vi "Navigation_florida_alex_rev0.vi"() -> ()   [LabVIEW 2015]
uses:
  <vilib>/myRIO/Instrument Drivers/Utilities/Utilities.lvlib
  <vilib>/rvi/interface/nirviReadWriteControl/nirviReadWriteControl.xnode
  NiFpgaLv.dll
  <vilib>/Utility/error.llb/Error Cluster From Error Code.vi
  <vilib>/rvi/interface/Simulation/niFpgaSimulationCallBeginRW.vi
  <vilib>/rvi/errors/niLvFpgaAdjustHostInterfaceError.vi
  <vilib>/rvi/interface/nirviOpenFPGA/nirviOpenFPGA.xnode
  FPGA Bitfiles/NavigationProjec_FPGATarget2_FPGAMainNavigati_PWPHW8gwDxI.lvbitx
  <vilib>/FPGAPlugInAG/myRIO-1900/niLvFpga_Open_myRIO-1900.vi
  <vilib>/rvi/interface/common/dynamic/niFpgaDynamicAddResources.vi
  <vilib>/myRIO/Instrument Drivers/Onboard IO/PWM/typedefs/PWM Configuration.ctl
  <vilib>/myRIO/Instrument Drivers/Onboard IO/PWM/PWM.lvlib
  <vilib>/myRIO/Common/Instrument Driver Framework/myRIO v1.0/PWM/typedefs/PWM Channels Enum.ctl
  <vilib>/myRIO/Common/Instrument Driver Framework/Utilities/typedefs/Generic FPGA Reference.ctl
  <vilib>/myRIO/Common/Instrument Driver Framework/Utilities/typedefs/myRIO v1.0 Reference.ctl
  <vilib>/myRIO/Common/Instrument Driver Framework/Utilities/typedefs/Hardware Version Enum.ctl
  <vilib>/myRIO/Common/Instrument Driver Framework/Utilities/typedefs/myRIO Generic Hardware Reference.ctl
  <vilib>/myRIO/Instrument Drivers/Onboard IO/PWM/typedefs/PWM Reference.ctl
  <vilib>/myRIO/Instrument Drivers/Onboard IO/PWM/vis/myRIO PWM Open.xnode
  <vilib>/myRIO/Common/Instrument Driver Framework/myRIO v1.0/PWM/vis/myRIO v1.1 Open PWM.vi
  <vilib>/userdefined/High Color/nirio_resource_hc.ctl
  <vilib>/addons/control/pid/NI_PID_pid.lvlib
  <vilib>/addons/control/pid/pid.llb/PID (DBL).vi
panel:
  in  "PID Gains Right":T1={"proportional gain (Kc)"=1.0, "integral time (Ti, min)"=0.01, "derivative time (Td, min)"=0.0} {"derivative time (Td, min)" format="%.3f"; "integral time (Ti, min)" format="%.3f"; "proportional gain (Kc)" format="%.3f"}
  in  "Output Range Right":cluster{"output high":dbl, "output low":dbl}={"output high"=100.0, "output low"=-100.0} {"output low" format="%.2f"; "output high" format="%.2f"}
  in  "Output Range Left":cluster{"output high":dbl, "output low":dbl}={"output high"=100.0, "output low"=-100.0} {"output low" format="%.2f"; "output high" format="%.2f"}
  in  "PID Gains Left":T1={"proportional gain (Kc)"=1.0, "integral time (Ti, min)"=0.01, "derivative time (Td, min)"=0.0} {"derivative time (Td, min)" format="%.3f"; "integral time (Ti, min)" format="%.3f"; "proportional gain (Kc)" format="%.3f"}
  out "Right Setpoint":dbl
  out "Left Setpoint":dbl
  out "Scale":dbl
  out "Distance to Goal":dbl
  out "Current Angle":dbl
  out "Current Y":dbl
  out "Current X":dbl
  out "State":i32
  out "Dump Angle":dbl
  out "Dump Y":dbl
  out "Dump X":dbl
  out "Start Case":i32
  out "Goal Y":dbl
  out "Goal X":dbl
  out "Start Angle":dbl
  out "Start Y":dbl
  out "Start X":dbl
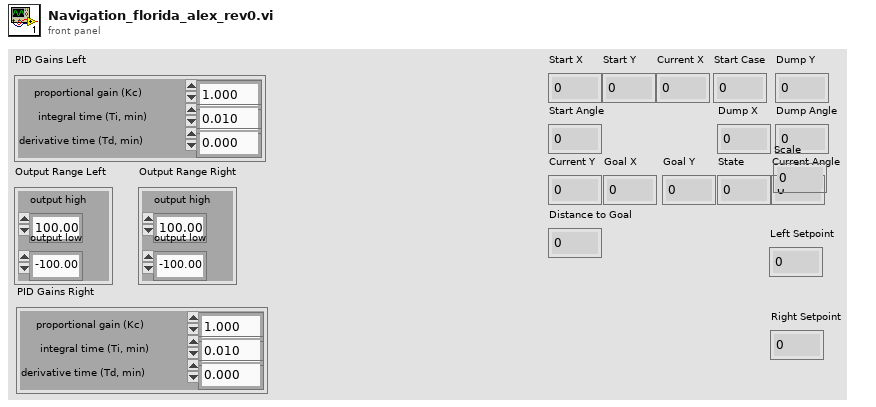
[diagram p1: front panel]
types:
  T1 = cluster{"proportional gain (Kc)":dbl, "integral time (Ti, min)":dbl, "derivative time (Td, min)":dbl}
  T2 = typedef "nirio_resource_hc.ctl" = tag
  T3 = typedef "Hardware Version Enum.ctl" = enum16{"Unknown", "myRIO-1900", "myRIO-1950", "roboRIO"}
  T4 = typedef "PWM.lvlib/PWM Reference.ctl" = cluster{"myRIO Reference":T5, "PWM Channels Enum":T8, "PWM Configuration":T9}
  T5 = typedef "myRIO Generic Hardware Reference.ctl" = cluster{"myRIO Model":T3, "myRIO Hardware Reference":T6}
  T6 = typedef "myRIO v1.0 Reference.ctl" = cluster{"Generic FPGA Reference":T7, "Allow multiple opens":bool}
  T7 = typedef "Generic FPGA Reference.ctl" = refnum<k20>
  T8 = typedef "PWM Channels Enum.ctl" = enum16{"Not Connected", "C/PWM0", "C/PWM1", "A/PWM0", "A/PWM1", "A/PWM2", "B/PWM0", "B/PWM1", "B/PWM2", "PWM/PWM0", "PWM/PWM1", "PWM/PWM2", "PWM/PWM3", "PWM/PWM4", "PWM/PWM5", "PWM/PWM6", "PWM/PWM7", "PWM/PWM8", "PWM/PWM9"}
  T9 = typedef "PWM.lvlib/PWM Configuration.ctl" = cluster{"Frequency":dbl, "Duty Cycle":dbl}
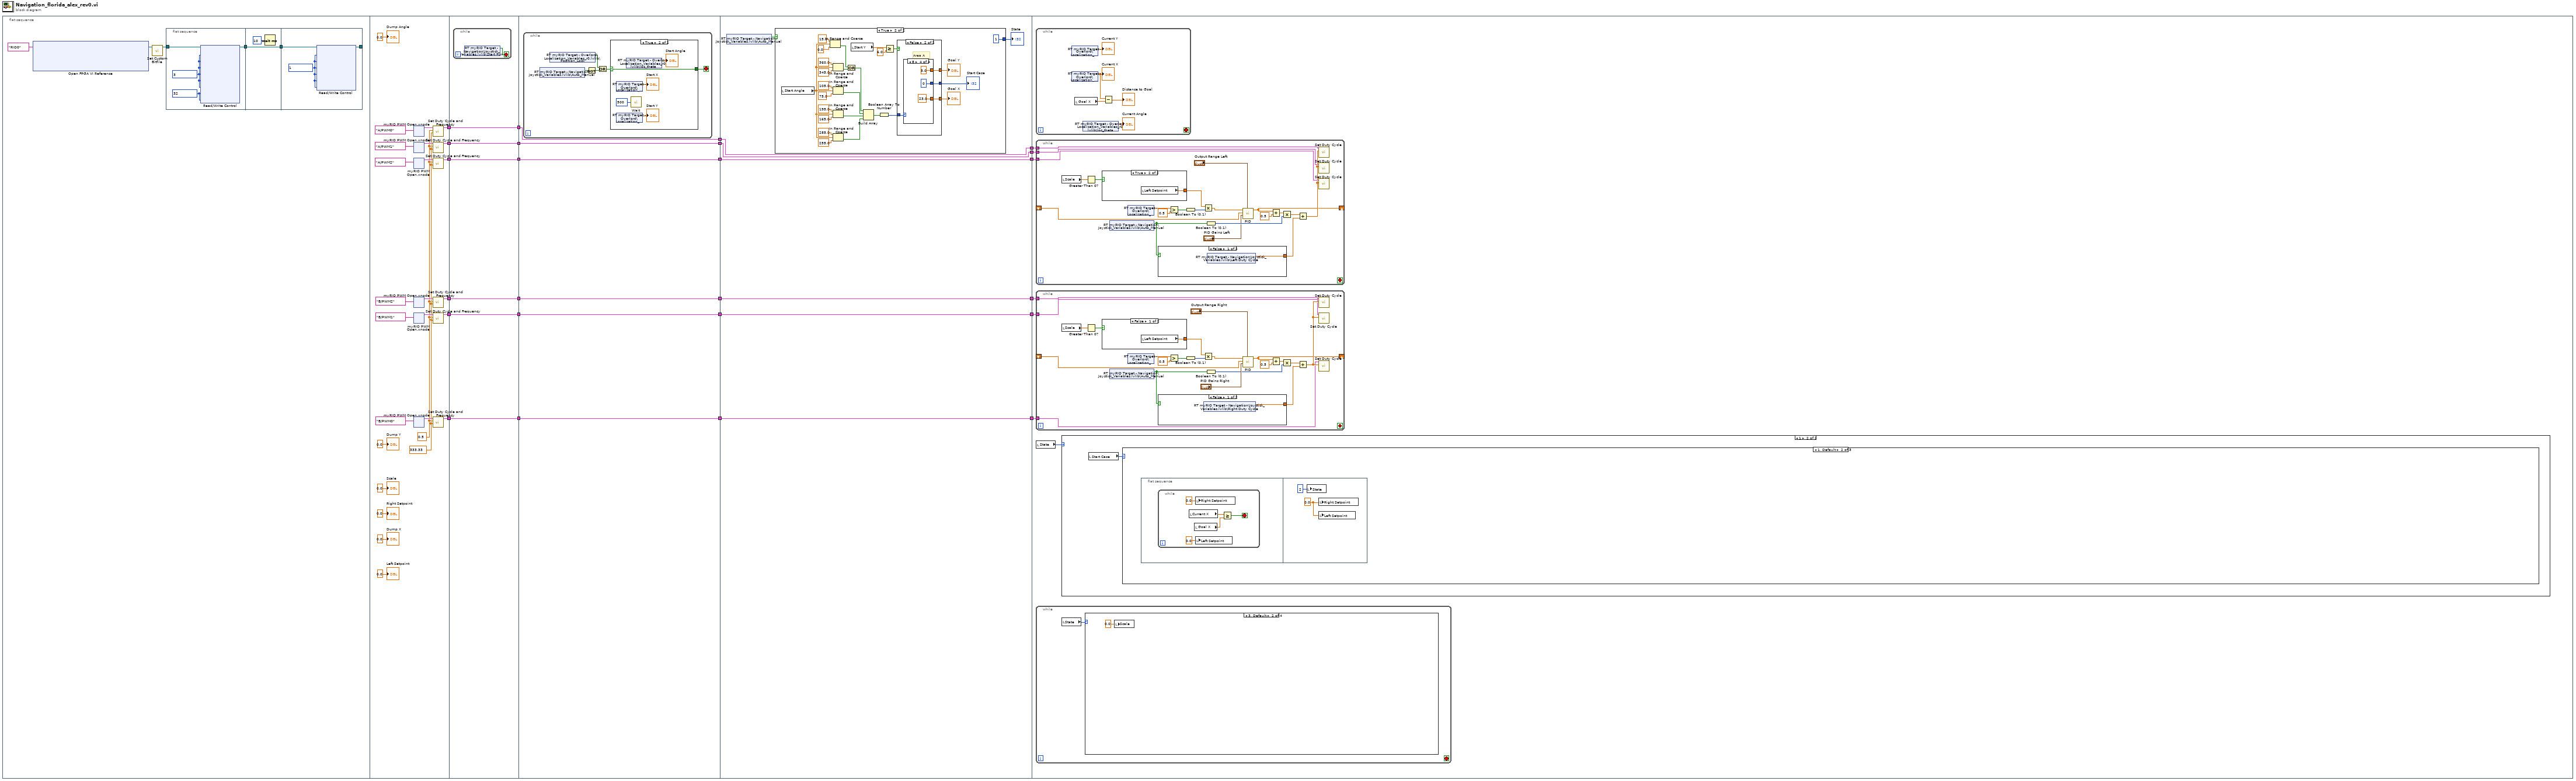
[diagram p0: block diagram]
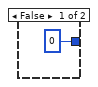
[diagram p3: hidden frame]
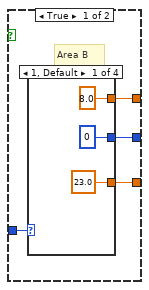
[diagram p4: hidden frame]
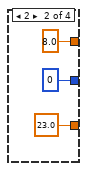
[diagram p5: hidden frame]
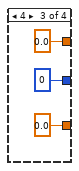
[diagram p6: hidden frame]
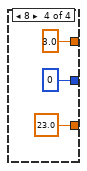
[diagram p7: hidden frame]
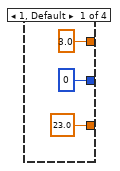
[diagram p8: hidden frame]
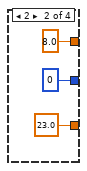
[diagram p9: hidden frame]
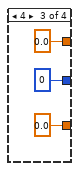
[diagram p10: hidden frame]
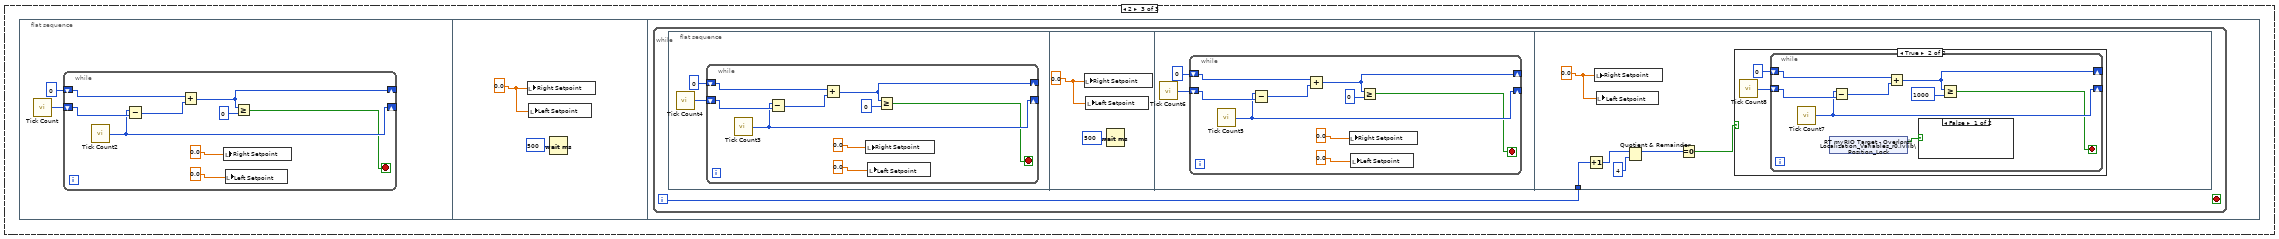
[diagram p13: hidden frame]
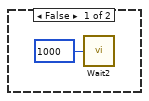
[diagram p14: hidden frame]
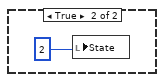
[diagram p15: hidden frame]
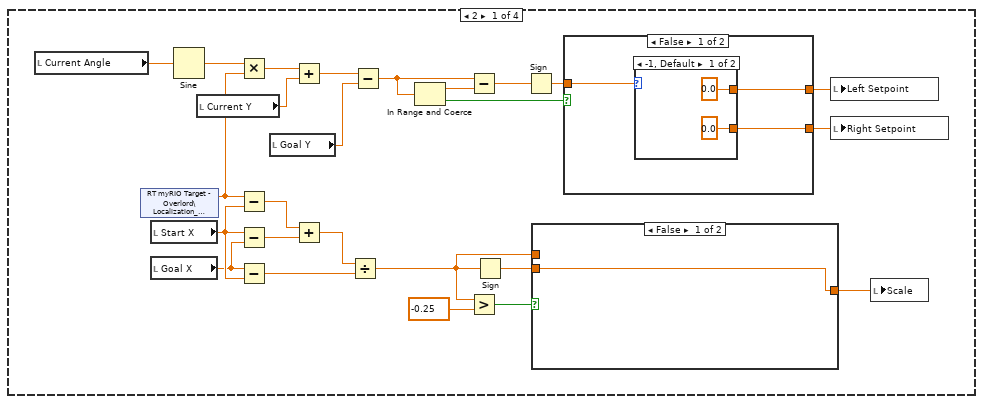
[diagram p16: hidden frame]
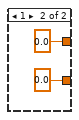
[diagram p17: hidden frame]
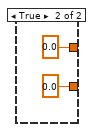
[diagram p18: hidden frame]
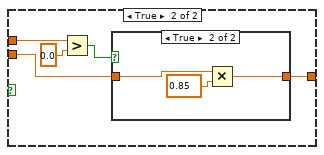
[diagram p19: hidden frame]
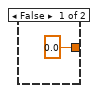
[diagram p20: hidden frame]
diagram:
  n1 = flat-sequence {
    tunnel: [w50] -> w24
    tunnel: [w49] -> w23
    tunnel: [w48] -> w22
    tunnel: [w47] -> w21
    tunnel: [w46] -> w20
    tunnel: [w45] -> w19
    tunnel: w24 -> [w166]
    tunnel: w23 -> [w165]
    tunnel: w22 -> [w164]
    tunnel: w21 -> [w163]
    tunnel: w20 -> [w162]
    tunnel: w19 -> [w161]
    tunnel: [w166] -> w18
    tunnel: [w165] -> w17
    tunnel: [w164] -> w16
    tunnel: [w163] -> w15
    tunnel: [w162] -> w14
    tunnel: [w161] -> w13
    tunnel: w18 -> [w173]
    tunnel: w17 -> [w172]
    tunnel: w16 -> [w171]
    tunnel: w15 -> [w170]
    tunnel: w14 -> [w169]
    tunnel: w13 -> [w168]
    tunnel: [w173] -> w12
    tunnel: [w172] -> w11
    tunnel: [w171] -> w10
    tunnel: [w170] -> w9
    tunnel: [w169] -> w8
    tunnel: [w168] -> w7
    tunnel: w12 -> [w192]
    tunnel: w11 -> [w191]
    tunnel: w10 -> [w190]
    tunnel: w9 -> [w189]
    tunnel: w8 -> [w188]
    tunnel: w7 -> [w187]
    tunnel: [w192] -> w6
    tunnel: [w191] -> w5
    tunnel: [w190] -> w4
    tunnel: [w189] -> w3
    tunnel: [w188] -> w2
    tunnel: [w187] -> w1
    tunnel: w6 -> [w258]
    tunnel: w5 -> [w257]
    tunnel: w4 -> [w256]
    tunnel: w3 -> [w255]
    tunnel: w2 -> [w254]
    tunnel: w1 -> [w253]
    frame #0 {
      n2 = xnode "Open FPGA VI Reference"("resource name"=tag "RIO0") -> ("FPGA VI Reference Out"=w26:refnum<k20>)  [unwired: 1 in, 1 out]
      n3 = call <vilib>:"Set Custom Bitfile.vi"("Custom FPGA Reference In"=w26) -> ("Custom FPGA Reference Out"=w27:refnum<k20>)  [unwired: 9 in, 1 out]
      n4 = flat-sequence {
        tunnel: w27 -> [w32]
        tunnel: [w30] -> w29
        tunnel: w29 -> [w34]
        tunnel: [w34] -> w28
        tunnel: w28 -> [w37]
        tunnel: [w36] -> _
        frame #0 {
          w31 = u8 32 ("SYS.SELECTA")
          w33 = u8 3 ("ENC.B_c.CNFG")
          n5 = xnode "Read/Write Control"("FPGA VI Reference In"=w32, "ENC.A_a.CNFG"=w33, "ENC.A_b.CNFG"=w33, "ENC.A_c.CNFG"=w33, "ENC.B_a.CNFG"=w33, "ENC.B_b.CNFG"=w33, "ENC.B_c.CNFG"=w33, "SYS.SELECTA"=w31, "SYS.SELECTB"=w31) -> ("FPGA VI Reference Out"=w30:refnum<k20>)  [unwired: 1 in, 1 out]
        }
        frame #1 {
          n6 = Wait (ms)(milliseconds to wait=u32 10) -> ()  [unwired: 1 out]
        }
        frame #2 {
          w38 = u8 1 ("ENC.B_c.CNFG")
          n7 = xnode "Read/Write Control"("FPGA VI Reference In"=w37, "ENC.A_a.CNFG"=w38, "ENC.A_b.CNFG"=w38, "ENC.A_c.CNFG"=w38, "ENC.B_a.CNFG"=w38, "ENC.B_b.CNFG"=w38, "ENC.B_c.CNFG"=w38) -> ("FPGA VI Reference Out"=w36:refnum<k20>)  [unwired: 1 in, 1 out]
        }
      }
    }
    frame #1 {
      w51 = 0.5
      w52 = 333.33
      n8 = xnode "myRIO PWM Open.xnode"("Channel Name"=tag "A/PWM0") -> ("PWM Ref Out"=w58:T4)  [unwired: 2 in, 1 out]
      n9 = xnode "myRIO PWM Open.xnode"("Channel Name"=tag "A/PWM1") -> ("PWM Ref Out"=w57:T4)  [unwired: 2 in, 1 out]
      n10 = xnode "myRIO PWM Open.xnode"("Channel Name"=tag "A/PWM2") -> ("PWM Ref Out"=w56:T4)  [unwired: 2 in, 1 out]
      n11 = xnode "myRIO PWM Open.xnode"("Channel Name"=tag "B/PWM2") -> ("PWM Ref Out"=w53:T4)  [unwired: 2 in, 1 out]
      n12 = xnode "myRIO PWM Open.xnode"("Channel Name"=tag "B/PWM1") -> ("PWM Ref Out"=w54:T4)  [unwired: 2 in, 1 out]
      n13 = xnode "myRIO PWM Open.xnode"("Channel Name"=tag "B/PWM0") -> ("PWM Ref Out"=w55:T4)  [unwired: 2 in, 1 out]
      n14 = call <vilib>:"Set Duty Cycle and Frequency.vi"("Frequency [Hz]"=w52, "Duty Cycle"=w51, "PWM Ref In"=w58) -> ("PWM Ref Out"=w50:T4)  [unwired: 6 in, 1 out]
      n15 = call <vilib>:"Set Duty Cycle and Frequency.vi"("Frequency [Hz]"=w52, "Duty Cycle"=w51, "PWM Ref In"=w57) -> ("PWM Ref Out"=w49:T4)  [unwired: 6 in, 1 out]
      n16 = call <vilib>:"Set Duty Cycle and Frequency.vi"("Frequency [Hz]"=w52, "Duty Cycle"=w51, "PWM Ref In"=w56) -> ("PWM Ref Out"=w48:T4)  [unwired: 6 in, 1 out]
      n17 = call <vilib>:"Set Duty Cycle and Frequency.vi"("Frequency [Hz]"=w52, "Duty Cycle"=w51, "PWM Ref In"=w53) -> ("PWM Ref Out"=w45:T4)  [unwired: 6 in, 1 out]
      n18 = call <vilib>:"Set Duty Cycle and Frequency.vi"("Frequency [Hz]"=w52, "Duty Cycle"=w51, "PWM Ref In"=w54) -> ("PWM Ref Out"=w46:T4)  [unwired: 6 in, 1 out]
      n19 = call <vilib>:"Set Duty Cycle and Frequency.vi"("Frequency [Hz]"=w52, "Duty Cycle"=w51, "PWM Ref In"=w55) -> ("PWM Ref Out"=w47:T4)  [unwired: 6 in, 1 out]
      "Dump X" <- 0.0
      "Dump Y" <- 0.0
      "Dump Angle" <- 0.0
      "Scale" <- 0.0
      "Left Setpoint" <- 0.0
      "Right Setpoint" <- 0.0
    }
    frame #2 {
      n20 = while {
        stop <- w167 stop-if-true
        n21 = shared-variable "RT myRIO Target - Navigation\\Joystick_Variables.lvlib\\Start Run"() -> (w167:bool)  [unwired: 1 in, 1 out]
      }
    }
    frame #3 {
      n22 = while {
        stop <- w174 stop-if-true
        n23 = shared-variable "RT myRIO Target - Navigation\\Joystick_Variables.lvlib\\Auto_Manual"() -> (w177:bool)  [unwired: 1 in, 1 out]
        n24 = shared-variable "RT myRIO Target - Overlord\\Localization_Variables_r0.lvlib\\Position_Lock"() -> (w178:bool)  [unwired: 1 in, 1 out]
        n25 = Not(x=w177) -> (.not. x?=w176:bool)
        n26 = Or(x=w178, y=w176) -> (x .or. y?=w175:bool)
        n27 = case shown="True" w175 {
          selector: w175 -> [w179 w181]
          tunnel: [w179 w181] -> w174
          frame False {
          }
          frame True {
            n28 = shared-variable "RT myRIO Target - Overlord\\Localization_Variables_r0.lvlib\\loc_x"() -> (→"Start X":dbl)  [unwired: 1 in, 1 out]
            n29 = shared-variable "RT myRIO Target - Overlord\\Localization_Variables_r0.lvlib\\loc_y"() -> (→"Start Y":dbl)  [unwired: 1 in, 1 out]
            n30 = shared-variable "RT myRIO Target - Overlord\\Localization_Variables_r0.lvlib\\loc_theta"() -> (→"Start Angle":dbl)  [unwired: 1 in, 1 out]
            n31 = call "Wait"("Count(mSec)"=u32 500) -> ()  [unwired: 1 out]
          }
        }
      }
    }
    frame #4 {
      n32 = shared-variable "RT myRIO Target - Navigation\\Joystick_Variables.lvlib\\Auto_Manual"() -> (w186:bool)  [unwired: 1 in, 1 out]
      n33 = case shown="True" w186 {
        tunnel: [0 1] -> w185
        frame False {
        }
        frame True {
          n34 = local read "Start Angle"() -> (w206:dbl)
          n35 = In Range and Coerce(upper limit=15.0, x=w206, lower limit=0.0) -> (In Range?=w205:bool)  [unwired: 1 out]
          n36 = In Range and Coerce(upper limit=360.0, x=w206, lower limit=345.0) -> (In Range?=w204:bool)  [unwired: 1 out]
          n37 = In Range and Coerce(upper limit=105.0, x=w206, lower limit=75.0) -> (In Range?=w202:bool)  [unwired: 1 out]
          n38 = In Range and Coerce(upper limit=195.0, x=w206, lower limit=165.0) -> (In Range?=w201:bool)  [unwired: 1 out]
          n39 = In Range and Coerce(upper limit=285.0, x=w206, lower limit=255.0) -> (In Range?=w200:bool)  [unwired: 1 out]
          n40 = Or(x=w205, y=w204) -> (x .or. y?=w203:bool)
          n41 = local read "Start Y"() -> (w219:dbl)
          n42 = Build Array(w203, w202, w201, w200) -> (w199:bool[])
          n43 = Boolean Array To Number(Boolean array=w199) -> (number=w198:u32)
          n44 = Greater Or Equal?(x=w219, y=6.0) -> (x >= y?=w217:bool)
          n45 = case shown="False" w217 {
            tunnel: w198 -> [w223 w239]
            tunnel: [w222 w238] -> w197
            tunnel: [w221 w237] -> w196
            tunnel: [w220 w236] -> w195
            frame True {
              # "Area B"
              n46 = case shown="1, Default" w223 {
                tunnel: [0 0 0 0] -> w220
                tunnel: [8.0 8.0 0.0 3.0] -> w221
                tunnel: [23.0 23.0 0.0 23.0] -> w222
                frame 1, Default {
                }
                frame 2 {
                }
                frame 4 {
                }
                frame 8 {
                }
              }
            }
            frame False {
              # "Area A"
              n47 = case shown="8" w239 {
                tunnel: [0 0 0 0] -> w236
                tunnel: [3.0 8.0 0.0 3.0] -> w237
                tunnel: [23.0 23.0 0.0 23.0] -> w238
                frame 1, Default {
                }
                frame 2 {
                }
                frame 4 {
                }
                frame 8 {
                }
              }
            }
          }
          "Goal X" <- w197
          "Goal Y" <- w196
          "Start Case" <- w195
        }
      }
      "State" <- w185
    }
    frame #5 {
      n48 = while {
        stop <- _ stop-if-true
        n49 = shared-variable "RT myRIO Target - Overlord\\Localization_Variables_r0.lvlib\\loc_y"() -> (→"Current Y":dbl)  [unwired: 1 in, 1 out]
        n50 = shared-variable "RT myRIO Target - Overlord\\Localization_Variables_r0.lvlib\\loc_x"() -> (w468:dbl)  [unwired: 1 in, 1 out]
        "Current X" <- w468
        n51 = local read "Goal X"() -> (w467:dbl)
        n52 = shared-variable "RT myRIO Target - Overlord\\Localization_Variables_r0.lvlib\\loc_theta"() -> (→"Current Angle":dbl)  [unwired: 1 in, 1 out]
        n53 = Subtract(x=w468, y=w467) -> (x-y=→"Distance to Goal":dbl)
      }
      n54 = while {
        tunnel: w258 -> [w447]
        tunnel: w257 -> [w446]
        tunnel: w256 -> [w445]
        shift-right: [w443] -> _
        shift-left: _ -> [w442]
        stop <- _ stop-if-true
        n55 = local read "Scale"() -> (w461:dbl)
        n56 = Greater Than 0?(x=w461) -> (x > 0?=w460:bool)
        n57 = case shown="True" w460 {
          tunnel: [w464 w465] -> w455
          frame False {
            n58 = local read "Right Setpoint"() -> (w464:dbl)
          }
          frame True {
            n59 = local read "Left Setpoint"() -> (w465:dbl)
          }
        }
        n60 = shared-variable "RT myRIO Target - Navigation\\Joystick_Variables.lvlib\\Auto_Manual"() -> (w459:bool)  [unwired: 1 in, 1 out]
        n61 = shared-variable "RT myRIO Target - Overlord\\Localization_Variables_r0.lvlib\\loc_x"() -> (w458:dbl)  [unwired: 1 in, 1 out]
        n62 = case shown="False" w459 {
          tunnel: [w462 0.0] -> w449
          frame False {
            n63 = shared-variable "RT myRIO Target - Navigation\\Joystick_Variables.lvlib\\Left Duty Cycle"() -> (w462:dbl)  [unwired: 1 in, 1 out]
          }
          frame True {
          }
        }
        n64 = Greater?(x=w458, y=0.5) -> (0:w456:bool)
        n65 = Boolean To (0,1)(Boolean=w456) -> (0, 1=w454:i16)
        n66 = Multiply(x=w455, y=w454) -> (x*y=w453:dbl)
        n67 = Boolean To (0,1)(Boolean=w459) -> (0, 1=w452:i16)
        n68 = call-poly <vilib>:"PID.vi"("output range"="Output Range Left", "PID gains"="PID Gains Left", "process variable"=w442, "setpoint"=w453) -> ("output"=w443:dbl)  [unwired: 6 in, 1 out]
        n69 = Add(x=w443, y=0.5) -> (x+y=w450:dbl)
        n70 = Multiply(x=w450, y=w452) -> (x*y=w448:dbl)
        n71 = Add(x=w448, y=w449) -> (x+y=w444:dbl)
        n72 = call <vilib>:"Set Duty Cycle.vi"("Duty Cycle"=w444, "PWM Ref In"=w447) -> ()  [unwired: 7 in, 2 out]
        n73 = call <vilib>:"Set Duty Cycle.vi"("Duty Cycle"=w444, "PWM Ref In"=w446) -> ()  [unwired: 7 in, 2 out]
        n74 = call <vilib>:"Set Duty Cycle.vi"("Duty Cycle"=w444, "PWM Ref In"=w445) -> ()  [unwired: 7 in, 2 out]
      }
      n75 = while {
        tunnel: w255 -> [w418]
        tunnel: w254 -> [w417]
        tunnel: w253 -> [w416]
        shift-right: [w415] -> _
        shift-left: _ -> [w414]
        stop <- _ stop-if-true
        n76 = local read "Scale"() -> (w435:dbl)
        n77 = Greater Than 0?(x=w435) -> (x > 0?=w434:bool)
        n78 = case shown="False" w434 {
          tunnel: [w438 w439] -> w430
          frame False {
            n79 = local read "Left Setpoint"() -> (w438:dbl)
          }
          frame True {
            n80 = local read "Right Setpoint"() -> (w439:dbl)
          }
        }
        n81 = shared-variable "RT myRIO Target - Navigation\\Joystick_Variables.lvlib\\Auto_Manual"() -> (w428:bool)  [unwired: 1 in, 1 out]
        n82 = shared-variable "RT myRIO Target - Overlord\\Localization_Variables_r0.lvlib\\loc_x"() -> (w431:dbl)  [unwired: 1 in, 1 out]
        n83 = case shown="False" w428 {
          tunnel: [w436 0.0] -> w420
          frame False {
            n84 = shared-variable "RT myRIO Target - Navigation\\Joystick_Variables.lvlib\\Right Duty Cycle"() -> (w436:dbl)  [unwired: 1 in, 1 out]
          }
          frame True {
          }
        }
        n85 = Greater?(x=w431, y=0.5) -> (0:w433:bool)
        n86 = Boolean To (0,1)(Boolean=w433) -> (0, 1=w429:i16)
        n87 = Multiply(x=w430, y=w429) -> (x*y=w427:dbl)
        n88 = Boolean To (0,1)(Boolean=w428) -> (0, 1=w422:i16)
        n89 = call-poly <vilib>:"PID.vi"("output range"="Output Range Right", "PID gains"="PID Gains Right", "process variable"=w414, "setpoint"=w427) -> ("output"=w415:dbl)  [unwired: 6 in, 1 out]
        n90 = Add(x=w415, y=0.5) -> (x+y=w423:dbl)
        n91 = Multiply(x=w423, y=w422) -> (x*y=w421:dbl)
        n92 = Add(x=w421, y=w420) -> (x+y=w419:dbl)
        n93 = call <vilib>:"Set Duty Cycle.vi"("Duty Cycle"=w419, "PWM Ref In"=w416) -> ()  [unwired: 7 in, 2 out]
        n94 = call <vilib>:"Set Duty Cycle.vi"("Duty Cycle"=w419, "PWM Ref In"=w417) -> ()  [unwired: 7 in, 2 out]
        n95 = call <vilib>:"Set Duty Cycle.vi"("Duty Cycle"=w419, "PWM Ref In"=w418) -> ()  [unwired: 7 in, 2 out]
      }
      n96 = local read "State"() -> (w252:i32)
      n97 = while {
        stop <- _ stop-if-true
        n98 = local read "State"() -> (w323:i32)
        n99 = case shown="3, Default" w323 {
          frame 2 {
            n100 = local read "Current Angle"() -> (w337:dbl)
            n101 = shared-variable "RT myRIO Target - Overlord\\Localization_Variables_r0.lvlib\\loc_x"() -> (w335:dbl)  [unwired: 1 in, 1 out]
            n102 = local read "Start X"() -> (w348:dbl)
            n103 = local read "Goal X"() -> (w347:dbl)
            n104 = Sine(x=w337) -> (sin(x)=w336:dbl)
            n105 = local read "Current Y"() -> (w333:dbl)
            n106 = Multiply(x=w336, y=w335) -> (x*y=w334:dbl)
            n107 = Subtract(x=w335, y=w348) -> (x-y=w346:dbl)
            n108 = Subtract(x=w348, y=w347) -> (x-y=w345:dbl)
            n109 = Subtract(x=w347, y=w348) -> (x-y=w344:dbl)
            n110 = local read "Goal Y"() -> (w332:dbl)
            n111 = Add(x=w334, y=w333) -> (x+y=w331:dbl)
            n112 = Add(x=w346, y=w345) -> (x+y=w343:dbl)
            n113 = Divide(x=w343, y=w344) -> (x/y=w340:dbl)
            n114 = Subtract(x=w331, y=w332) -> (x-y=w328:dbl)
            n115 = In Range and Coerce(x=w328) -> (coerced(x)=w329:dbl, In Range?=w330:bool)  [unwired: 2 in]
            n116 = Subtract(x=w328, y=w329) -> (x-y=w327:dbl)
            n117 = Greater?(x=w340, y=-0.25) -> (0:w341:bool)
            n118 = Sign(1:w340) -> (0:w339:dbl)
            n119 = Sign(1:w327) -> (0:w326:dbl)
            n120 = case shown="False" w341 {
              tunnel: w340 -> [_ w362]
              tunnel: w339 -> [w358 w360]
              tunnel: [w358 w359] -> w338
              frame False {
              }
              frame True {
                n121 = Greater?(x=w362, y=0.0) -> (0:w361:bool)
                n122 = case shown="True" w361 {
                  tunnel: w360 -> [_ w367]
                  tunnel: [0.0 w365] -> w359
                  frame False {
                  }
                  frame True {
                    n123 = Multiply(x=w367, y=0.85) -> (x*y=w365:dbl)
                  }
                }
              }
            }
            n124 = case shown="False" w330 {
              tunnel: w326 -> [w351 _]
              tunnel: [w350 0.0] -> w324
              tunnel: [w349 0.0] -> w325
              frame False {
                n125 = case shown="-1, Default" w351 {
                  tunnel: [0.0 0.0] -> w350
                  tunnel: [0.0 0.0] -> w349
                  frame -1, Default {
                  }
                  frame 1 {
                  }
                }
              }
              frame True {
              }
            }
            n126 = local write "Left Setpoint"(w325) -> ()
            n127 = local write "Right Setpoint"(w324) -> ()
            n128 = local write "Scale"(w338) -> ()
          }
          frame 3, Default {
            n129 = local write "Scale"(0.0) -> ()
          }
          frame 4 {
            n130 = local read "Current Angle"() -> (w382:dbl)
            n131 = shared-variable "RT myRIO Target - Overlord\\Localization_Variables_r0.lvlib\\loc_x"() -> (w380:dbl)  [unwired: 1 in, 1 out]
            n132 = local read "Start X"() -> (w393:dbl)
            n133 = local read "Goal X"() -> (w392:dbl)
            n134 = Sine(x=w382) -> (sin(x)=w381:dbl)
            n135 = local read "Current Y"() -> (w378:dbl)
            n136 = Multiply(x=w381, y=w380) -> (x*y=w379:dbl)
            n137 = Subtract(x=w380, y=w393) -> (x-y=w391:dbl)
            n138 = Subtract(x=w393, y=w392) -> (x-y=w390:dbl)
            n139 = Subtract(x=w392, y=w393) -> (x-y=w389:dbl)
            n140 = local read "Goal Y"() -> (w377:dbl)
            n141 = Add(x=w379, y=w378) -> (x+y=w376:dbl)
            n142 = Add(x=w391, y=w390) -> (x+y=w388:dbl)
            n143 = Divide(x=w388, y=w389) -> (x/y=w385:dbl)
            n144 = Subtract(x=w376, y=w377) -> (x-y=w373:dbl)
            n145 = In Range and Coerce(x=w373) -> (coerced(x)=w374:dbl, In Range?=w375:bool)  [unwired: 2 in]
            n146 = Subtract(x=w373, y=w374) -> (x-y=w372:dbl)
            n147 = Greater?(x=w385, y=-0.25) -> (0:w386:bool)
            n148 = Sign(1:w385) -> (0:w384:dbl)
            n149 = Sign(1:w372) -> (0:w371:dbl)
            n150 = case shown="False" w386 {
              tunnel: w385 -> [_ w407]
              tunnel: w384 -> [w403 w405]
              tunnel: [w403 w404] -> w383
              frame False {
              }
              frame True {
                n151 = Greater?(x=w407, y=0.0) -> (0:w406:bool)
                n152 = case shown="True" w406 {
                  tunnel: w405 -> [_ w412]
                  tunnel: [0.0 w410] -> w404
                  frame False {
                  }
                  frame True {
                    n153 = Multiply(x=w412, y=0.85) -> (x*y=w410:dbl)
                  }
                }
              }
            }
            n154 = case shown="False" w375 {
              tunnel: w371 -> [w396 _]
              tunnel: [w395 0.0] -> w369
              tunnel: [w394 0.0] -> w370
              frame False {
                n155 = case shown="-1, Default" w396 {
                  tunnel: [0.0 0.0] -> w395
                  tunnel: [0.0 0.0] -> w394
                  frame -1, Default {
                  }
                  frame 1 {
                  }
                }
              }
              frame True {
              }
            }
            n156 = local write "Left Setpoint"(w370) -> ()
            n157 = local write "Right Setpoint"(w369) -> ()
            n158 = local write "Scale"(w383) -> ()
          }
          frame 5 {
            n159 = local write "Scale"(0.0) -> ()
          }
        }
      }
      n160 = case shown="1" w252 {
        frame 0, Default {
        }
        frame 1 {
          n161 = local read "Start Case"() -> (w259:i32)
          n162 = case shown="1, Default" w259 {
            frame 0 {
            }
            frame 1, Default {
              n163 = flat-sequence {
                frame #0 {
                  n164 = while {
                    stop <- w262 stop-if-true
                    n165 = local read "Current X"() -> (w263:dbl)
                    n166 = local read "Goal X"() -> (w264:dbl)
                    n167 = local write "Right Setpoint"(0.0) -> ()
                    n168 = local write "Left Setpoint"(0.0) -> ()
                    n169 = Greater Or Equal?(x=w263, y=w264) -> (x >= y?=w262:bool)
                  }
                }
                frame #1 {
                  w265 = 0.0
                  n170 = local write "State"(2) -> ()
                  n171 = local write "Right Setpoint"(w265) -> ()
                  n172 = local write "Left Setpoint"(w265) -> ()
                }
              }
            }
            frame 2 {
              n173 = flat-sequence {
                frame #0 {
                  n174 = call "Tick Count"() -> ("Tick Count(mSec)"=w267:u32)
                  n175 = while {
                    shift-right: [w272] -> _
                    shift-left: 0 -> [w277]
                    shift-right: [w274] -> _
                    shift-left: w267 -> [w276]
                    stop <- w271 stop-if-true
                    n176 = call "Tick Count2"() -> ("Tick Count(mSec)"=w274:u32)
                    n177 = Subtract(x=w274, y=w276) -> (x-y=w275:u32)
                    n178 = Add(x=w277, y=w275) -> (x+y=w272:u32)
                    n179 = local write "Right Setpoint"(0.0) -> ()
                    n180 = local write "Left Setpoint"(0.0) -> ()
                    n181 = Greater Or Equal?(x=w272, y=u32 0) -> (x >= y?=w271:bool)
                  }
                }
                frame #1 {
                  w279 = 0.0
                  n182 = local write "Right Setpoint"(w279) -> ()
                  n183 = local write "Left Setpoint"(w279) -> ()
                  n184 = Wait (ms)(milliseconds to wait=u32 500) -> ()  [unwired: 1 out]
                }
                frame #2 {
                  n185 = while {
                    i -> [w280]
                    stop <- _ stop-if-true
                    n186 = flat-sequence {
                      tunnel: w280 -> [w309]
                      frame #0 {
                        n187 = call "Tick Count4"() -> ("Tick Count(mSec)"=w282:u32)
                        n188 = while {
                          shift-right: [w286] -> _
                          shift-left: 0 -> [w291]
                          shift-right: [w288] -> _
                          shift-left: w282 -> [w290]
                          stop <- w285 stop-if-true
                          n189 = call "Tick Count3"() -> ("Tick Count(mSec)"=w288:u32)
                          n190 = Subtract(x=w288, y=w290) -> (x-y=w289:u32)
                          n191 = Add(x=w291, y=w289) -> (x+y=w286:u32)
                          n192 = local write "Right Setpoint"(0.0) -> ()
                          n193 = local write "Left Setpoint"(0.0) -> ()
                          n194 = Greater Or Equal?(x=w286, y=u32 0) -> (x >= y?=w285:bool)
                        }
                      }
                      frame #1 {
                        w292 = 0.0
                        n195 = local write "Right Setpoint"(w292) -> ()
                        n196 = local write "Left Setpoint"(w292) -> ()
                        n197 = Wait (ms)(milliseconds to wait=u32 500) -> ()  [unwired: 1 out]
                      }
                      frame #2 {
                        n198 = call "Tick Count6"() -> ("Tick Count(mSec)"=w294:u32)
                        n199 = while {
                          shift-right: [w299] -> _
                          shift-left: 0 -> [w304]
                          shift-right: [w301] -> _
                          shift-left: w294 -> [w303]
                          stop <- w298 stop-if-true
                          n200 = call "Tick Count5"() -> ("Tick Count(mSec)"=w301:u32)
                          n201 = Subtract(x=w301, y=w303) -> (x-y=w302:u32)
                          n202 = Add(x=w304, y=w302) -> (x+y=w299:u32)
                          n203 = local write "Right Setpoint"(0.0) -> ()
                          n204 = local write "Left Setpoint"(0.0) -> ()
                          n205 = Greater Or Equal?(x=w299, y=u32 0) -> (x >= y?=w298:bool)
                        }
                      }
                      frame #3 {
                        w310 = 0.0
                        n206 = Increment(x=w309) -> (x+1=w308:i32)
                        n207 = local write "Right Setpoint"(w310) -> ()
                        n208 = local write "Left Setpoint"(w310) -> ()
                        n209 = Quotient & Remainder(x=w308, y=4) -> (x-y*floor(x/y)=w306:i32)  [unwired: 1 out]
                        n210 = Equal To 0?(x=w306) -> (x = 0?=w305:bool)
                        n211 = case shown="True" w305 {
                          frame False {
                            n212 = call "Wait2"("Count(mSec)"=u32 1000) -> ()  [unwired: 1 out]
                          }
                          frame True {
                            n213 = call "Tick Count8"() -> ("Tick Count(mSec)"=w313:u32)
                            n214 = while {
                              shift-right: [w316] -> _
                              shift-left: 0 -> [w321]
                              shift-right: [w318] -> _
                              shift-left: w313 -> [w320]
                              stop <- w315 stop-if-true
                              n215 = call "Tick Count7"() -> ("Tick Count(mSec)"=w318:u32)
                              n216 = shared-variable "RT myRIO Target - Overlord\\Localization_Variables_r0.lvlib\\Position_Lock"() -> (w314:bool)  [unwired: 1 in, 1 out]
                              n217 = Subtract(x=w318, y=w320) -> (x-y=w319:u32)
                              n218 = Add(x=w321, y=w319) -> (x+y=w316:u32)
                              n219 = case shown="False" w314 {
                                frame False {
                                }
                                frame True {
                                n220 = local write "State"(2) -> ()
                                }
                              }
                              n221 = Greater Or Equal?(x=w316, y=u32 1000) -> (x >= y?=w315:bool)
                            }
                          }
                        }
                      }
                    }
                  }
                }
              }
            }
          }
        }
      }
    }
  }
